vi "A-K_meas.vi"(11 "Input wave":waveform(dbl)) -> (0 "Katod_dbl":T1, 1 "Katod_str":T3, 2 "Anod_dbl":T2, 3 "Anod_str":T4)   [LabVIEW 2012]
uses:
  <vilib>/Analysis/5stat.llb/RMS (DBL).vi
  <vilib>/Analysis/baseanly.llb/Mean (DBL).vi
  <vilib>/Analysis/NI_AALPro.lvlib
  <vilib>/Analysis/NI_AALBase.lvlib
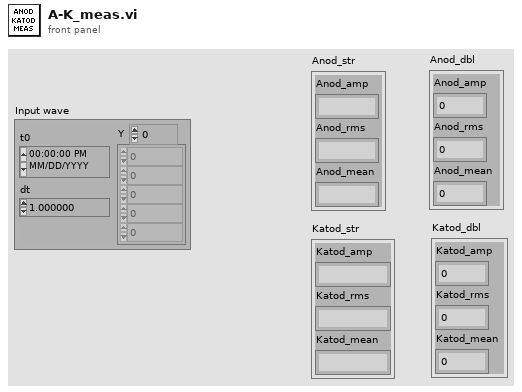
[diagram p1: front panel]
types:
  T1 = cluster{"Katod_amp":dbl, "Katod_rms":dbl, "Katod_mean":dbl}
  T2 = cluster{"Anod_amp":dbl, "Anod_rms":dbl, "Anod_mean":dbl}
  T3 = cluster{"Katod_amp":string, "Katod_rms":string, "Katod_mean":string}
  T4 = cluster{"Anod_amp":string, "Anod_rms":string, "Anod_mean":string}
  T5 = cluster{string, "rms value":string, "mean":string}
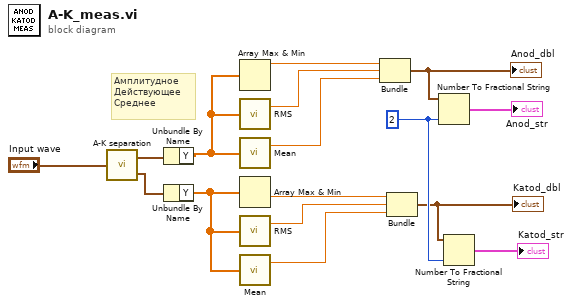
[diagram p0: block diagram]
diagram:
  w3 = i16 2 ("precision (6)")
  # "Амплитудное\nДействующее \nСреднее"
  n1 = call "A-K separation.vi"("Input wave"="Input wave") -> ("Katod wave (inverted)"=w14:waveform(dbl), "Anod wave"=w13:waveform(dbl))  [unwired: 3 in]
  n2 = Unbundle By Name(w13) -> ("Y"=w15:dbl[])
  n3 = Unbundle By Name(w14) -> ("Y"=w16:dbl[])
  n4 = Array Max & Min(array=w15) -> (max value=w11:dbl)  [unwired: 3 out]
  n5 = call-poly <vilib>:"RMS.vi"("X"=w15) -> ("rms value"=w10:dbl)  [unwired: 1 out]
  n6 = call-poly <vilib>:"Mean.vi"("X"=w15) -> ("mean"=w9:dbl)  [unwired: 1 out]
  n7 = Array Max & Min(array=w16) -> (min value=w6:dbl)  [unwired: 3 out]
  n8 = call-poly <vilib>:"RMS.vi"("X"=w16) -> ("rms value"=w5:dbl)  [unwired: 1 out]
  n9 = call-poly <vilib>:"Mean.vi"("X"=w16) -> ("mean"=w4:dbl)  [unwired: 1 out]
  n10 = Bundle(w11, "rms value"=w10, "mean"=w9) -> (w8:cluster{dbl, "rms value":dbl, "mean":dbl})  [unwired: 1 in]
  "Anod_dbl" <- w8
  n11 = Bundle(w6, "rms value"=w5, "mean"=w4) -> (w1:cluster{dbl, "rms value":dbl, "mean":dbl})  [unwired: 1 in]
  "Katod_dbl" <- w1
  n12 = Number To Fractional String(number=w8, precision (6)=w3) -> (F-format string=→"Anod_str":T5)  [unwired: 2 in]
  n13 = Number To Fractional String(number=w1, precision (6)=w3) -> (F-format string=→"Katod_str":T5)  [unwired: 2 in]
